vi "Parse DelayFormula.vi"(8 "error in (no error)":errorcluster, 9 "DelayFormula":string, 10 "BME_DG_System":refnum<class "BME_DG_System.lvclass">, 11 "BME_DG_Chnl in":refnum<class "BME_DG_Chnl.lvclass">) -> (0 "error out":errorcluster, 1 "Problem Chnls out":string[](array[string]), 2 "BME_DG_System out":refnum<class "BME_DG_System.lvclass">)   [LabVIEW 2009, in "POLARIS BME DG.lvlib" / "BME_DG_Chnl.lvclass"]
uses:
  BME_DG_Chnl.lvclass
  BME_DG_System/BME_DG_System.lvclass
  BME_DG_Chnl.lvclass/BME_DG_Chnl.ctl
  <vilib>/gmath/NI_Gmath.lvlib
  POLARIS BME DG.lvlib
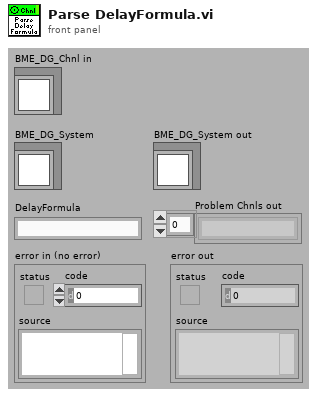
[diagram p1: front panel]
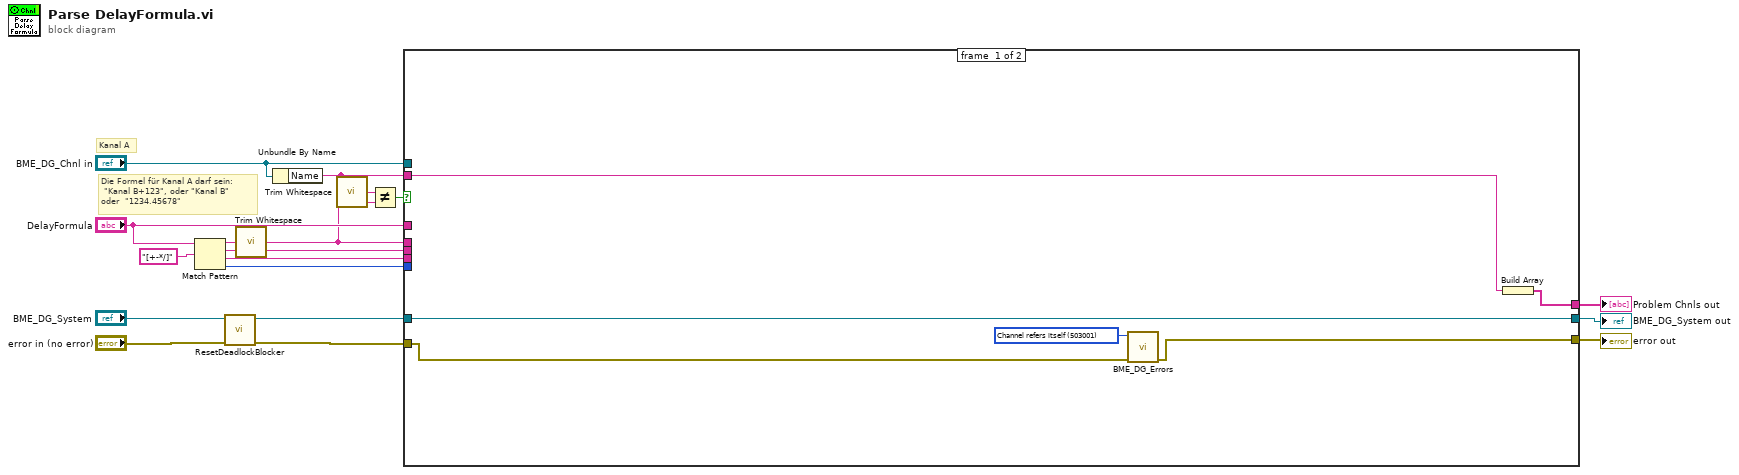
[diagram p0: block diagram]
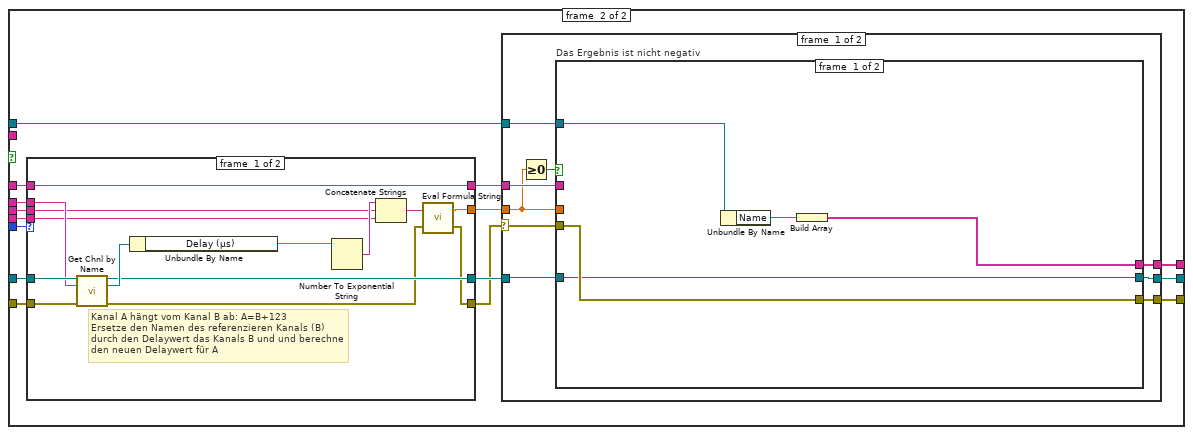
[diagram p2: hidden frame]
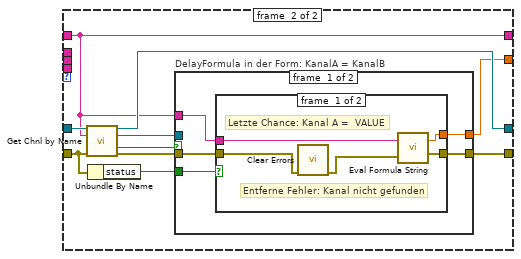
[diagram p3: hidden frame]
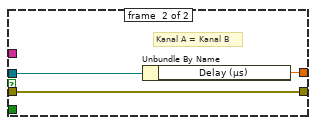
[diagram p5: hidden frame]
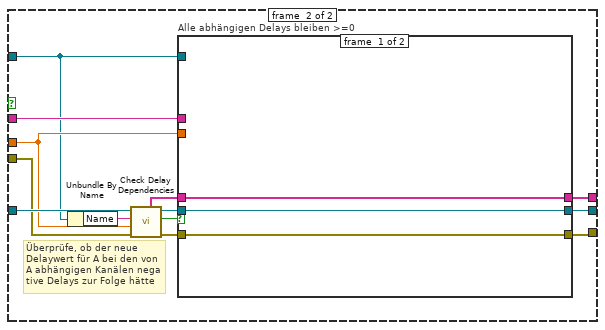
[diagram p6: hidden frame]
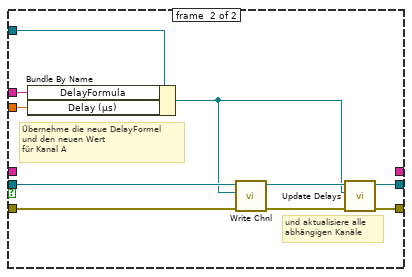
[diagram p7: hidden frame]
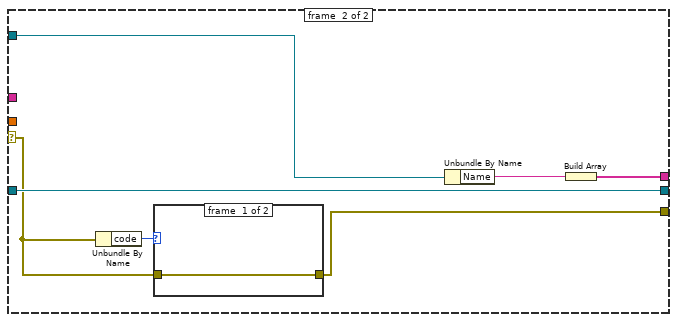
[diagram p8: hidden frame]
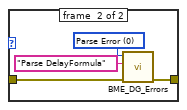
[diagram p9: hidden frame]
diagram:
  # "Die Formel für Kanal A darf sein:\n \"Kanal B+123\", oder \"Kanal B\" \noder  \"1234.45678\""
  # "Kanal A"
  n1 = Match Pattern(string="DelayFormula", regular expression="[+-*/]") -> (before substring=w17:string, match substring=w12:string, after substring=w11:string, offset past match=w13:i32)  [unwired: 1 in]
  n2 = call "ResetDeadlockBlocker.vi"("error in (no error)"="error in (no error)", "BME_DG_System in"="BME_DG_System") -> ("error out"=w1:errorcluster, "BME_DG_System out"=w3:refnum<class "BME_DG_System.lvclass">)  [unwired: 8 in]
  n3 = call <vilib>:"Trim Whitespace.vi"("string"=w17) -> ("trimmed string"=w6:string)  [unwired: 1 in]
  n4 = Unbundle By Name("BME_DG_Chnl in") -> ("Name"=w5:string)
  n5 = call <vilib>:"Trim Whitespace.vi"("string"=w5) -> ("trimmed string"=w7:string)  [unwired: 1 in]
  n6 = Not Equal?(x=w7, y=w6) -> (x != y?=w8:bool)
  n7 = case shown="True" w8 {
    tunnel: w1 -> [w20 w39]
    tunnel: "BME_DG_Chnl in" -> [_ w38]
    tunnel: w3 -> [w24 w37]
    tunnel: w6 -> [_ w36]
    tunnel: [w19 w34] -> w16
    tunnel: [w22 w33] -> w15
    tunnel: [w24 w32] -> w14
    tunnel: w13 -> [_ w31]
    tunnel: w12 -> [_ w30]
    tunnel: w11 -> [_ w29]
    tunnel: "DelayFormula" -> [_ w28]
    tunnel: w5 -> [w23 _]
    frame #0 {
      w21 = 503001 items=["Channel refers itself"=503001, "Deadloop"=503002, "Negative Delay"=503003] ("error")
      n8 = call "BME_DG_Errors.vi"("error in (no error)"=w20, "error"=w21) -> ("error out"=w19:errorcluster)  [unwired: 9 in]
      n9 = Build Array(w23) -> (w22:string[])
    }
    frame #1 {
      n10 = case shown="-1" w31 {
        tunnel: w39 -> [w53 w55]
        tunnel: w37 -> [w52 w63]
        tunnel: w36 -> [w50 _]
        tunnel: [w40 w60] -> w25
        tunnel: [w49 w62] -> w35
        tunnel: w30 -> [w46 _]
        tunnel: w29 -> [w45 _]
        tunnel: w28 -> [w44 w61]
        tunnel: [w44 w61] -> w27
        tunnel: [w41 w58] -> w26
        frame #0 {
          # "Kanal A hängt vom Kanal B ab: A=B+123\nErsetze den Namen des referenzieren Kanals (B)\ndurch den Delaywert das Kanals B und und berechne \nden neuen Delaywert für A"
          n11 = call "Get Chnl by Name.vi"("BME_DG_System in"=w52, "Chnl Name"=w50, "error in (no error)"=w53) -> ("BME_DG_System out"=w49:refnum<class "BME_DG_System.lvclass">, "BME_DG_Chnl"=w51:refnum<class "BME_DG_Chnl.lvclass">, "error out"=w42:errorcluster)  [unwired: 7 in, 3 out]
          n12 = Unbundle By Name(w51) -> ("Delay (µs)"=w48:dbl)
          n13 = Number To Exponential String(number=w48) -> (E-format string=w47:string)  [unwired: 3 in]
          n14 = Concatenate Strings(w47, w46, w45) -> (w43:string)
          n15 = call <vilib>:"Eval Formula String.vi"("error in (no error)"=w42, "formula"=w43) -> ("error out"=w40:errorcluster, "y value"=w41:dbl)
        }
        frame #1 {
          n16 = call "Get Chnl by Name.vi"("BME_DG_System in"=w63, "Chnl Name"=w61, "error in (no error)"=w55) -> ("BME_DG_System out"=w62:refnum<class "BME_DG_System.lvclass">, "BME_DG_Chnl"=w59:refnum<class "BME_DG_Chnl.lvclass">, "found?"=w57:bool, "error out"=w56:errorcluster)  [unwired: 7 in, 2 out]
          n17 = Unbundle By Name(w55) -> ("status"=w54:bool)
          n18 = case "DelayFormula in der Form: KanalA = KanalB" shown="False" w57 {
            tunnel: w61 -> [w68 _]
            tunnel: [w66 w75] -> w60
            tunnel: w59 -> [_ w77]
            tunnel: [w67 w76] -> w58
            tunnel: w56 -> [w65 w75]
            tunnel: w54 -> [w64 _]
            frame #0 {
              n19 = case shown="False" w64 {
                tunnel: w68 -> [w73 _]
                tunnel: [w72 _] -> w67
                tunnel: [w71 w74] -> w66
                tunnel: w65 -> [w70 w74]
                frame #0 {
                  # "Entferne Fehler: Kanal nicht gefunden"
                  # "Letzte Chance: Kanal A =  VALUE"
                  n20 = call <vilib>:"Clear Errors.vi"("error in (no error)"=w70) -> ("error out"=w69:errorcluster)  [unwired: 6 in]
                  n21 = call <vilib>:"Eval Formula String.vi"("error in (no error)"=w69, "formula"=w73) -> ("error out"=w71:errorcluster, "y value"=w72:dbl)
                }
                frame #1 {
                }
              }
            }
            frame #1 {
              # "Kanal A = Kanal B"
              n22 = Unbundle By Name(w77) -> ("Delay (µs)"=w76:dbl)
            }
          }
        }
      }
      n23 = case shown="No Error" w25 {
        selector: w25 -> [w81 w119]
        tunnel: w38 -> [w86 w124]
        tunnel: w27 -> [w85 _]
        tunnel: w26 -> [w83 _]
        tunnel: w35 -> [w82 w121]
        tunnel: [w80 w118] -> w34
        tunnel: [w79 w122] -> w33
        tunnel: [w78 w121] -> w32
        frame #0 {
          n24 = Greater Or Equal To 0?(x=w83) -> (x >= 0?=w84:bool)
          n25 = case "Das Ergebnis ist nicht negativ" shown="True" w84 {
            tunnel: w86 -> [w91 w99]
            tunnel: w85 -> [_ w104]
            tunnel: w83 -> [_ w100]
            tunnel: w82 -> [w87 w103]
            tunnel: w81 -> [w88 w101]
            tunnel: [w88 w92] -> w80
            tunnel: [w89 w96] -> w79
            tunnel: [w87 w98] -> w78
            frame #0 {
              n26 = Unbundle By Name(w91) -> ("Name"=w90:string)
              n27 = Build Array(w90) -> (w89:string[])
            }
            frame #1 {
              # "Überprüfe, ob der neue\nDelaywert für A bei den von \nA abhängigen Kanälen nega\ntive Delays zur Folge hätte"
              n28 = Unbundle By Name(w99) -> ("Name"=w93:string)
              n29 = call "Check Delay Dependencies.vi"("error in (no error)"=w101, "new Delay"=w100, "Chnl"=w93, "BME_DG_System in"=w103) -> ("error out"=w94:errorcluster, "Dependecies OK"=w102:bool, "BME_DG_System out"=w97:refnum<class "BME_DG_System.lvclass">, "Problem Chnls out"=w95:string[])  [unwired: 4 in]
              n30 = case "Alle abhängigen Delays bleiben >=0" shown="True" w102 {
                tunnel: w99 -> [_ w117]
                tunnel: w104 -> [_ w116]
                tunnel: w100 -> [_ w115]
                tunnel: [w107 w114] -> w98
                tunnel: w97 -> [w107 w112]
                tunnel: [w105 _] -> w96
                tunnel: w95 -> [w105 _]
                tunnel: w94 -> [w106 w110]
                tunnel: [w106 w113] -> w92
                frame #0 {
                }
                frame #1 {
                  # "und aktualisiere alle\nabhängigen Kanäle"
                  # "Übernehme die neue DelayFormel\nund den neuen Wert\nfür Kanal A"
                  n31 = Bundle By Name(cluster=w117, "DelayFormula"=w116, "Delay (µs)"=w115) -> (w108:refnum<class "BME_DG_Chnl.lvclass">)
                  n32 = call "Write Chnl.vi"("error in (no error)"=w110, "BME_DG_Chnl.lvclass"=w108, "BME_DG_System in"=w112) -> ("error out"=w109:errorcluster, "BME_DG_System out"=w111:refnum<class "BME_DG_System.lvclass">)  [unwired: 7 in]
                  n33 = call "Update Delays.vi"("error in (no error)"=w109, "BME_DG_Chnl in"=w108, "BME_DG_System in"=w111) -> ("error out"=w113:errorcluster, "BME_DG_System out"=w114:refnum<class "BME_DG_System.lvclass">)  [unwired: 7 in]
                }
              }
            }
          }
        }
        frame #1 {
          n34 = Unbundle By Name(w119) -> ("code"=w120:i32)
          n35 = case shown="-23087" w120 {
            tunnel: w119 -> [w125 w129]
            tunnel: [w125 w128] -> w118
            frame #0 {
            }
            frame #1 {
              w127 = 0 items=["Channel refers itself"=503001, "Deadloop"=503002, "Negative Delay"=503003, "Delay Card not found"=503004, "Channel not found"=503005, "Parse Error"=0] ("error")
              n36 = call "BME_DG_Errors.vi"("error in (no error)"=w129, "source"="Parse DelayFormula", "error"=w127) -> ("error out"=w128:errorcluster)  [unwired: 8 in]
            }
          }
          n37 = Unbundle By Name(w124) -> ("Name"=w123:string)
          n38 = Build Array(w123) -> (w122:string[])
        }
      }
    }
  }
  "error out" <- w16
  "Problem Chnls out" <- w15
  "BME_DG_System out" <- w14
